vi "Get Configuration settings.vi"(6 "error in (no error)":errorcluster, 9 "File path":T3={"configuration"=path "c:/Parametros.cfg", "confRFID"=path "c:/RFID/TAGS.csv", "LOG.txt"=path "", "Path LOG"=path "c:/TEST", "Path_data"=path "c:/Trenes", "TAGS leidos"=path "c:/RFID/TAGS.csv", "configuracion flota"=path "", "flota"=path "", "Nombre de archivo"=[], "Folder calibration"=path "", "calibration log"=path "", "Reporting Procesamiento"=path "", "Error ejes"=path "", "Reporting Adquisición"=path ""}) -> (0 "error out":errorcluster, 1 "output cluster":T4, 3 "Cfg":T1={"RFID NEM on?"=FALSE, "RFID LR6 on?"=FALSE, "Use Aura?"=FALSE, "Leer config RFID NEM"=FALSE, "Canal cero WS1?"=FALSE, "Canal cero WS2 "=FALSE, "Digital?"=TRUE, "Reset watchdog?"=FALSE, "Able watchdog?"=FALSE, "Borrar archivos\nadquisicion con error"=FALSE, "AURA wheel test"=FALSE, "Save calibration"=FALSE, "Puerto RFID"=2189, "Port LR6"=2001, "timeout ms (60000)"=0, "bytes to read"=0, "DeviceAddress"=0, "IP RFID"="192.168.106.99", "IP synchr"="", "LR6 IP address"="192.168.106.94", "Parametros AuraWheel"=[], "Frecuencia de muestreo y módulo CRIO"=2, "Escaneos de la FIFO por canal"=5000, "Frecuencia de muestreo (Hz)"=25600.0, "dt RMS"=256.0, "Tiempo extra al detector de paso (s)"=1.0, "Count(mSec)"=2, "Offset_rueda WS 1"=0.004999998956918716, "Offset_rueda WS 2"=0.004999998956918716, "Nº de acelerómetros"=0, "Nº inductivos"=0, "Max archivos"=2, "Bytes min libre"=2, "Bytes libre despues de borrar"=2, "Timeout ruedas"=0.0, "Pattern amplitude (g)"=1.02, "Pattern frequency (Hz)"=159.2, "Tiempo de adquisicion\n"=10.0, "Parámetros acelerómetros"=[], "Inicio pasada"=timestamp(0 s since 1904-01-01), "Ultimo TEST"=timestamp(0 s since 1904-01-01), "Report_AURA"="", "Temperatura (ºC)"=0.0, "Direccion 0?"=FALSE} {"Offset_rueda WS 2" format="%.27g"; "Offset_rueda WS 1" format="%.27g"; "Frecuencia de muestreo y módulo CRIO" items=["51.200 kS/s (NI 9234)"=1, "25.600 kS/s (NI 9234)"=2, "17.067 kS/s (NI 9234)"=3, "12.800 kS/s (NI 9234)"=4, "10.240 kS/s (NI 9234)"=5, "8.533 kS/s (NI 9234)"=6, "7.314 kS/s (NI 9234)"=7, "6.400 kS/s (NI 9234)"=8, "5.689 kS/s (NI 9234)"=9, "5.120 kS/s (NI 9234)"=10, "4.654 kS/s (NI 9234)"=11, "4.267 kS/s (NI 9234)"=12, "3.938 kS/s (NI 9234)"=13, "3.657 kS/s (NI 9234)"=14, "3.413 kS/s (NI 9234)"=15, "3.200 kS/s (NI 9234)"=16, "3.012 kS/s (NI 9234)"=17, "2.845 kS/s (NI 9234)"=18, "2.695 kS/s (NI 9234)"=19, "2.560 kS/s (NI 9234)"=20, "2.438 kS/s (NI 9234)"=21, "2.328 kS/s (NI 9234)"=22, "2.226 kS/s (NI 9234)"=23, "2.133 kS/s (NI 9234)"=24, "2.048 kS/s (NI 9234)"=25, "1.969 kS/s (NI 9234)"=26, "1.896 kS/s (NI 9234)"=27, "1.829 kS/s (NI 9234)"=28, "1.765 kS/s (NI 9234)"=29, "1.707 kS/s (NI 9234)"=30, "1.652 kS/s (NI 9234)"=31]})   [LabVIEW 2015]
doc: "Obtain parameters from Parametros.cfg and set passing time"
uses:
  controls/File paths.ctl
  controls/Cfg_parameters.ctl
  <vilib>/LabVIEW Targets/FPGA/cRIO/shared/nicrio_ModuleControls/nicrio_cRIO-9234_DataRatesRing2.ctl
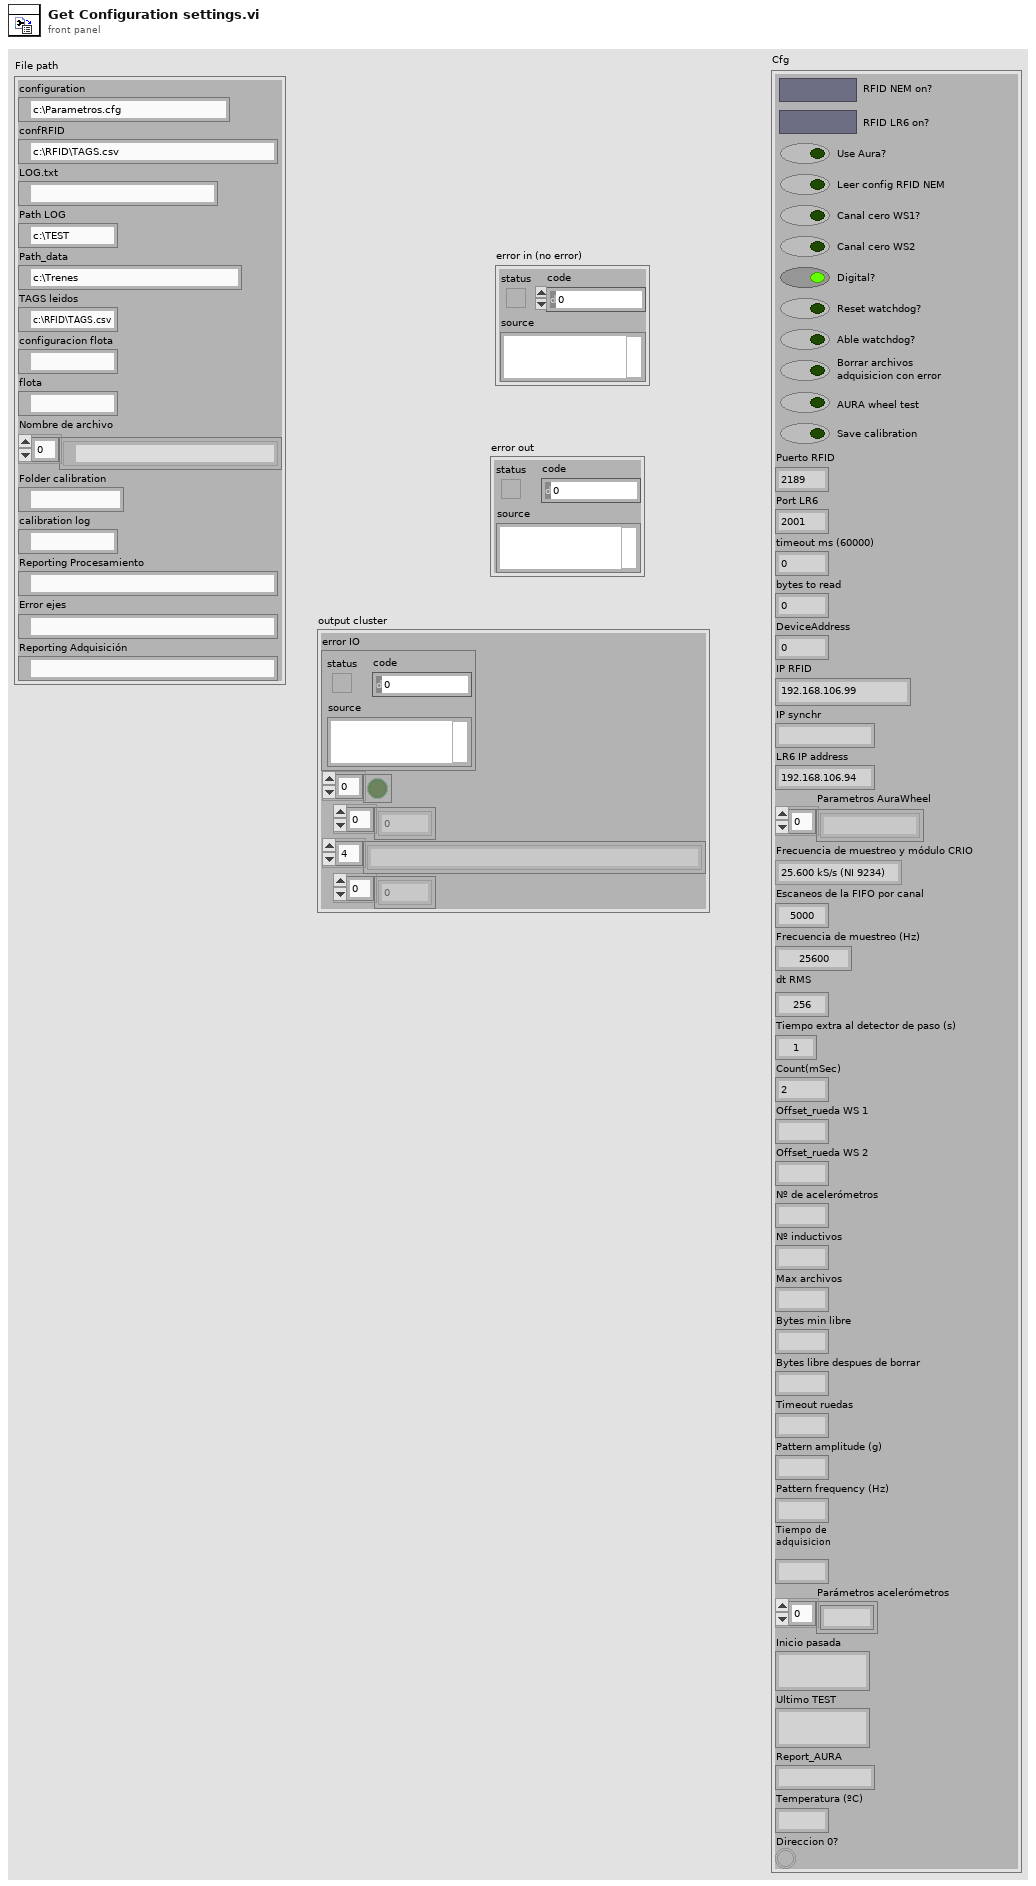
[diagram p1: front panel]
types:
  T1 = typedef "Cfg_parameters.ctl" = cluster{"RFID NEM on?":bool, "RFID LR6 on?":bool, "Use Aura?":bool, "Leer config RFID NEM":bool, "Canal cero WS1?":bool, "Canal cero WS2 ":bool, "Digital?":bool, "Reset watchdog?":bool, "Able watchdog?":bool, "Borrar archivos\nadquisicion con error":bool, "AURA wheel test":bool, "Save calibration":bool, "Puerto RFID":u16, "Port LR6":u16, "timeout ms (60000)":i32, "bytes to read":i32, "DeviceAddress":u8, "IP RFID":string, "IP synchr":string, "LR6 IP address":string, "Parametros AuraWheel":string[], "Frecuencia de muestreo y módulo CRIO":T2, "Escaneos de la FIFO por canal":u32, "Frecuencia de muestreo (Hz)":dbl, "dt RMS":dbl, "Tiempo extra al detector de paso (s)":dbl, "Count(mSec)":u32, "Offset_rueda WS 1":fxp<+/-,24,-4>, "Offset_rueda WS 2":fxp<+/-,24,-4>, "Nº de acelerómetros":i32, "Nº inductivos":i32, "Max archivos":u32, "Bytes min libre":u32, "Bytes libre despues de borrar":u32, "Timeout ruedas":dbl, "Pattern amplitude (g)":dbl, "Pattern frequency (Hz)":dbl, "Tiempo de adquisicion\n":dbl, "Parámetros acelerómetros":dbl[], "Inicio pasada":timestamp, "Ultimo TEST":timestamp, "Report_AURA":string, "Temperatura (ºC)":dbl, "Direccion 0?":bool}
  T2 = typedef "nicrio_cRIO-9234_DataRatesRing2.ctl" = u8
  T3 = typedef "File paths.ctl" = cluster{"configuration":path, "confRFID":path, "LOG.txt":path, "Path LOG":path, "Path_data":path, "TAGS leidos":path, "configuracion flota":path, "flota":path, "Nombre de archivo":path[], "Folder calibration":path, "calibration log":path, "Reporting Procesamiento":path, "Error ejes":path, "Reporting Adquisición":path}
  T4 = cluster{"error IO":errorcluster, bool[], u32[], string[], dbl[]}
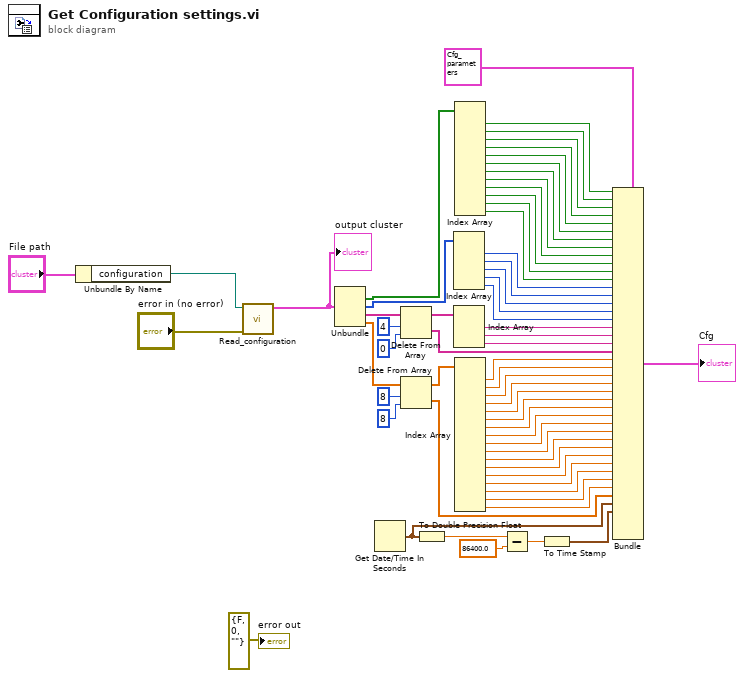
[diagram p0: block diagram]
diagram:
  n1 = Unbundle By Name("File path") -> ("configuration"=w4:path)
  n2 = call "Read_configuration.vi"("error in (no error)"="error in (no error)", "configuration file path"=w4) -> ("output cluster"=w11:T4)  [unwired: 8 in, 1 out]
  "output cluster" <- w11
  n3 = Unbundle(w11) -> (w60:bool[], w46:u32[], w39:string[], w29:dbl[])  [unwired: 1 out]
  n4 = Get Date/Time In Seconds() -> (seconds since 1Jan1904=w6:timestamp)
  n5 = Delete From Array(array=w39, length=4, index=0) -> (deleted portion=w38:string[], array with subset deleted=w41:string[])
  n6 = Delete From Array(array=w29, length=8, index=8) -> (deleted portion=w30:dbl[], array with subset deleted=w33:dbl[])
  n7 = To Double Precision Float(number=w6) -> (double precision float=w9:dbl)
  n8 = Index Array(array=w46) -> (element #1=w47:u32, element #2=w45:u32, element #3=w44:u32, element #4=w43:u32, element #5=w42:u32)  [unwired: 5 in]
  n9 = Index Array(array=w41) -> (element #1=w36:string, element #2=w35:string, element #3=w34:string)  [unwired: 3 in]
  n10 = Index Array(array=w60) -> (element #1=w59:bool, element #2=w58:bool, element #3=w57:bool, element #4=w56:bool, element #5=w55:bool, element #6=w50:bool, element #7=w49:bool, element #8=w48:bool, element #9=w51:bool, element #10=w52:bool, element #11=w53:bool, element #12=w54:bool)  [unwired: 12 in]
  n11 = Index Array(array=w33) -> (element #1=w28:dbl, element #2=w27:dbl, element #3=w26:dbl, element #4=w25:dbl, element #5=w24:dbl, element #6=w23:dbl, element #7=w22:dbl, element #8=w21:dbl, element #9=w20:dbl, element #10=w19:dbl, element #11=w18:dbl, element #12=w17:dbl, element #13=w16:dbl, element #14=w15:dbl, element #15=w14:dbl, element #16=w13:dbl, element #17=w12:dbl)  [unwired: 17 in]
  n12 = Subtract(x=w9, y=86400.0) -> (x-y=w8:dbl)
  n13 = To Time Stamp(1:w8) -> (0:w7:timestamp)
  n14 = Bundle(cluster=T1 {"RFID NEM on?"=FALSE, "RFID LR6 on?"=FALSE, "Use Aura?"=FALSE, "Leer config RFID NEM"=FALSE, "Canal cero WS1?"=FALSE, "Canal cero WS2 "=FALSE, "Digital?"=TRUE, "Reset watchdog?"=FALSE, "Able watchdog?"=FALSE, "Borrar archivos\nadquisicion con error"=FALSE, "AURA wheel test"=FALSE, "Save calibration"=FALSE, "Puerto RFID"=2189, "Port LR6"=2001, "timeout ms (60000)"=0, "bytes to read"=0, "DeviceAddress"=0, "IP RFID"="192.168.106.99", "IP synchr"="", "LR6 IP address"="192.168.106.94", "Parametros AuraWheel"=[], "Frecuencia de muestreo y módulo CRIO"=2, "Escaneos de la FIFO por canal"=5000, "Frecuencia de muestreo (Hz)"=25600.0, "dt RMS"=256.0, "Tiempo extra al detector de paso (s)"=1.0, "Count(mSec)"=2, "Offset_rueda WS 1"=0.004999998956918716, "Offset_rueda WS 2"=0.004999998956918716, "Nº de acelerómetros"=0, "Nº inductivos"=0, "Max archivos"=2, "Bytes min libre"=2, "Bytes libre despues de borrar"=2, "Timeout ruedas"=0.0, "Pattern amplitude (g)"=1.02, "Pattern frequency (Hz)"=159.2, "Tiempo de adquisicion\n"=10.0, "Parámetros acelerómetros"=[], "Inicio pasada"=timestamp(0 s since 1904-01-01), "Ultimo TEST"=timestamp(0 s since 1904-01-01), "Report_AURA"="", "Temperatura (ºC)"=0.0, "Direccion 0?"=FALSE} ("Cfg"), "RFID NEM on?"=w59, "RFID LR6 on?"=w58, "Use Aura?"=w57, "Leer config RFID NEM"=w56, "Canal cero WS1?"=w55, "Canal cero WS2"=w50, "Digital?"=w49, "Reset watchdog?"=w48, "Able watchdog?"=w51, "Borrar archivos\nadquisicion con error"=w52, "AURA wheel test"=w53, "Save calibration"=w54, "Puerto RFID"=w47, "Port LR6"=w45, "timeout ms (60000)"=w44, "bytes to read"=w43, "DeviceAddress"=w42, "IP RFID"=w36, "IP synchr"=w35, "LR6 IP address"=w34, "Parametros AuraWheel"=w38, "Frecuencia de muestreo y módulo CRIO"=w28, "Escaneos de la FIFO por canal"=w27, "Frecuencia de muestreo (Hz)"=w26, "dt RMS"=w25, "Tiempo extra al detector de paso (s)"=w24, "Count(mSec)"=w23, "Offset_rueda WS 1"=w22, "Offset_rueda WS 2"=w21, "Nº de acelerómetros"=w20, "Nº inductivos"=w19, "Max archivos"=w18, "Bytes min libre"=w17, "Bytes libre despues de borrar"=w16, "Timeout ruedas"=w15, "Pattern amplitude (g)"=w14, "Pattern frequency (Hz)"=w13, "Tiempo de adquisicion"=w12, "Parámetros acelerómetros"=w30, "Inicio pasada"=w6, "Ultimo TEST"=w7) -> (→"Cfg":T1)  [unwired: 3 in]
  "error out" <- errorcluster {"status"=FALSE, "code"=0, "source"=""} ("error out")
